vi "SetDataEventCreatorName.vi"(8 "error in (no error)":errorcluster, 10 "data event creator":string) -> (0 "error out":errorcluster)   [LabVIEW 2017, in "GlobalConfiguration.lvlib"]
uses:
  <vilib>/addons/InsightCM/Utilities/GlobalConfiguration/GlobalConfiguration.lvlib
  <vilib>/addons/PointValueMap/subVIs/Point_Write_string.vi
  <vilib>/addons/PointValueMap/PointValueMap.lvlib
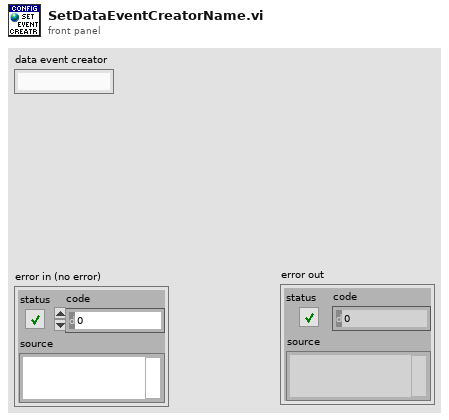
[diagram p1: front panel]
types:
  T1 = typedef "PointValueMap.lvlib/PointMap.ctl" = refnum<data-value>
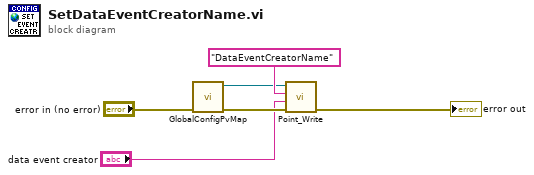
[diagram p0: block diagram]
diagram:
  n1 = call <vilib>:"GlobalConfigPvMap.vi"("error in (no error)"="error in (no error)") -> ("error out"=w3:errorcluster, "global configuration map"=w4:T1)  [unwired: 9 in]
  n2 = call-poly <vilib>:"Point_Write.vi"("Error In"=w3, "Value"="data event creator", "Tag"="DataEventCreatorName" ("Name"), "Map"=w4) -> ("Error Out"=→"error out":errorcluster)  [unwired: 6 in, 1 out]
